vi "modify channel test.vi"() -> (0 "no err":errorcluster, 3 "mod success":bool)   [LabVIEW 2015, in "Sequencer Module tests.lvlib"]
doc: "Tests the 'Replace Line' VI."
uses:
  Sequencer Module tests.lvlib
  <vilib>/NI/Tag Bus Module Framework/channel/TBM channel.lvclass/TBM channel.ctl
  <vilib>/NI/Tag Bus Module Framework/channel/channel classification.ctl
  <vilib>/NI/Tag Bus/tag/tag descriptor.lvclass/tag descriptor.ctl
  <vilib>/NI/Tag Bus Module Framework/channel/Read channel classification.vi
  <vilib>/NI/Tag Bus Module Framework/channel/Write channel classification.vi
  module/configuration/Sequencer Module configuration.lvclass
  <vilib>/NI/Tag Bus Module Framework/channel/TBM channel.lvclass
  <vilib>/NI/Tag Bus/tag/tag descriptor.lvclass
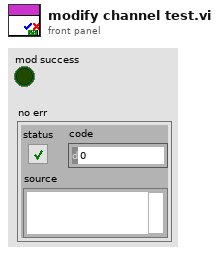
[diagram p1: front panel]
types:
  T1 = typedef "Sequencer Module configuration.lvclass/Line.ctl" = cluster{"channel":refnum<class "TBM channel.lvclass">}
  T2 = typedef "TBM channel.lvclass/channel classification.ctl" = enum16{"input data", "output data", "processing parameter", "processing result"}
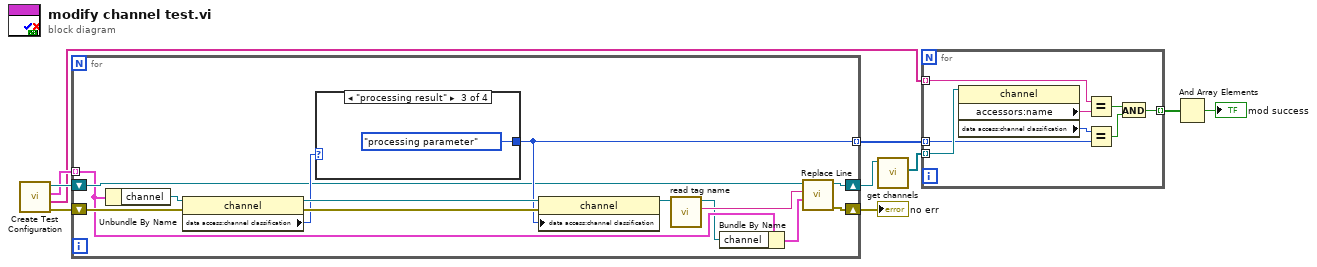
[diagram p0: block diagram]
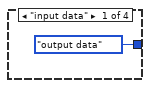
[diagram p2: hidden frame]
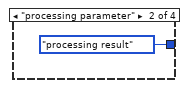
[diagram p3: hidden frame]
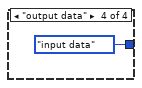
[diagram p4: hidden frame]
diagram:
  n1 = call "Create Test Configuration.vi"() -> ("error out"=w2:errorcluster, "Names"=w1:string[], "Line Array"=w3:T1[], "Module Configuration"=w4:refnum<class "Sequencer Module configuration.lvclass">)  [unwired: 6 in, 2 out]
  n2 = for {
    shift-right: [w17] -> w10
    shift-left: w4 -> [w16]
    shift-right: [w18] -> w9
    shift-left: w2 -> [w24]
    tunnel: w3 -> [w15] mode=indexing
    tunnel: [w20] -> w5 mode=indexing
    n3 = Unbundle By Name(w15) -> ("channel"=w19:refnum<class "TBM channel.lvclass">)
    n4 = property class="channel"(reference=w19, error in=w24) -> (reference out=w22:refnum<class "TBM channel.lvclass">, error out=w23:errorcluster, "data access:channel classification"=w21:T2)
    n5 = case shown="\"processing result\"" w21 {
      tunnel: [channel_classification."output data" ("channel classification") channel_classification."processing result" ("channel classification") channel_classification."processing parameter" ("channel classification") channel_classification."input data" ("channel classification")] -> w20
      frame "input data" {
      }
      frame "processing parameter" {
      }
      frame "processing result" {
      }
      frame "output data" {
      }
    }
    n6 = property class="channel"(reference=w22, error in=w23, "data access:channel classification"=w20) -> (reference out=w12:refnum<class "TBM channel.lvclass">)  [unwired: 1 out]
    n7 = call <vilib>:"read tag name.vi"("system tag in"=w12) -> ("name"=w13:string, "system tag out"=w11:refnum<class "TBM channel.lvclass">)  [unwired: 8 in, 1 out]
    n8 = Bundle By Name(cluster=w15, "channel"=w11) -> (w14:T1)
    n9 = call "Replace Line.vi"("New Line"=w14, "Line Name"=w13, "Sequencer Module configuration in"=w16) -> ("error out"=w18:errorcluster, "Sequencer Module configuration out"=w17:refnum<class "Sequencer Module configuration.lvclass">)  [unwired: 6 in, 1 out]
  }
  "no err" <- w9
  n10 = call-dynamic "get channels.vi"("Sequencer Module configuration in"=w10) -> ("channels"=w8:refnum<class "TBM channel.lvclass">[])  [unwired: 9 in, 1 out]
  n11 = for {
    tunnel: w8 -> [w35] mode=indexing
    tunnel: [w34] -> w7 mode=indexing
    tunnel: w5 -> [w33] mode=indexing
    tunnel: w1 -> [w30] mode=indexing
    n12 = property class="channel"(reference=w35) -> ("accessors:name"=w31:string, "data access:channel classification"=w32:T2)  [unwired: 1 in, 2 out]
    n13 = Equal?(x=w30, y=w31) -> (x = y?=w29:bool)
    n14 = Equal?(x=w32, y=w33) -> (x = y?=w36:bool)
    n15 = And(x=w29, y=w36) -> (x .and. y?=w34:bool)
  }
  n16 = And Array Elements(Boolean array=w7) -> (logical AND=→"mod success":bool)
